vi "Lat Long Conversion.vi"   [LabVIEW 2014]
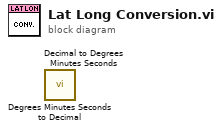
[diagram p0: block diagram]
diagram:
  n1 = call "Degrees Minutes Seconds to Decimal.vi"() -> ()  [unwired: 11 in, 1 out]
  n2 = call "Decimal to Degrees Minutes Seconds.vi"() -> ()  [unwired: 9 in, 3 out]
